vi "_io_write_with_OPC_synchro.vi"(4 "Send *ESR? at the end (T)":bool=TRUE, 5 "Attribute":T1={"Identifier"="", "Descriptive Name"="", "Data Type"=enum."Integer 32", "Command"="", "Access"=enum."Read/Write", "Range Table"="", "Read Callback"="", "Write Callback"="", "Supported Models"="", "Instrument Options"="", "Index"=0, "OPC Wait"=FALSE, "No Status Check"=FALSE, "Cache Only"=FALSE}, 7 "Timeout in (0 = OPC timeout)":i32, 8 "error in":errorcluster caption="error in (no error)", 10 "Write Command":string, 11 "VISA resource name":refnum<visa-resource-name>) -> (0 "error out":errorcluster, 2 "OPC Waited":bool, 3 "VISA resource name out":refnum<visa-resource-name>)   [LabVIEW 2020, in "Rohde&Schwarz RTx Oscilloscopes.lvlib" / "rsidr_core.lvlib"]
uses:
  rsidr_core.lvlib
  type_Attribute.ctl
  type_Attribute_Data_Type.ctl
  type_ReadWriteAccess.ctl
  whitespace.ctl
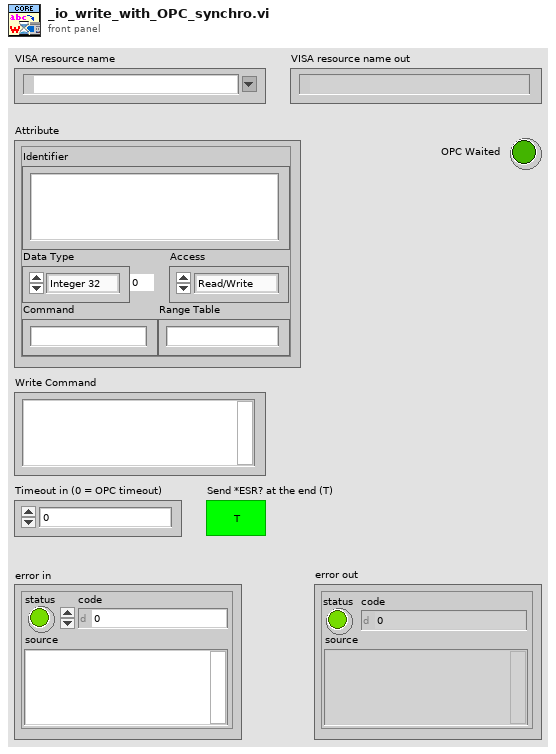
[diagram p1: front panel]
types:
  T1 = typedef "Rohde&Schwarz RTx Oscilloscopes.lvlib/rsidr_core.lvlib/type_Attribute.ctl" = cluster{"Identifier":string, "Descriptive Name":string, "Data Type":T2, "Command":string, "Access":T3, "Range Table":string, "Read Callback":string, "Write Callback":string, "Supported Models":string, "Instrument Options":string, "Index":i32, "OPC Wait":bool, "No Status Check":bool, "Cache Only":bool}
  T2 = typedef "Rohde&Schwarz RTx Oscilloscopes.lvlib/rsidr_core.lvlib/type_Attribute_Data_Type.ctl" = enum16{"Integer 32", "Double", "String", "Boolean", "None", "Integer 64", "RawString"}
  T3 = typedef "Rohde&Schwarz RTx Oscilloscopes.lvlib/rsidr_core.lvlib/type_ReadWriteAccess.ctl" = enum16{"Read Only", "Write Only", "Read/Write"}
  T4 = typedef "Rohde&Schwarz RTx Oscilloscopes.lvlib/rsidr_core.lvlib/type_Session_Data.ctl" = cluster{"IDN string":string, "Instrument FW":string, "Instr type":string, "Instr type for err. msg.":string, "Installed Options":string[], "Ignore Error Messages":string, "Logging params":variant, "OPC Timeout":i32, "VISA Timeout":i32, "STB Poll VISA Timeout":i32, "Additional Flags":i32, "Wait Before Read":i32, "Wait Before Write":i32, "Option String Flags":i32, "IO Segment Size":i64, "VISA Access Mode":T5, "Interface Type":T6, "OPC Wait Mode":T7, "Bin Float Number  Format":T8, "Bin Integer Number Format":T9, "Simulate":bool, "VXIcapable":bool, "Duplicate Session":bool, "Add LF to Write":bool, "Logging":bool, "Fast Sweep":bool, "Query Instrument Status":bool, "Check Range":bool, "Check Options":bool, "OPC-sync Attr Writes":bool, "OPC-sync Attr Queries":bool}
  T5 = typedef "Rohde&Schwarz RTx Oscilloscopes.lvlib/rsidr_core.lvlib/type_VisaAccessMode.ctl" = u16
  T6 = typedef "Rohde&Schwarz RTx Oscilloscopes.lvlib/rsidr_core.lvlib/type_InterfaceType.ctl" = enum16{"Unknown", "GPIB", "VXI", "GPIB_VXI", "ASRL", "PXI", "TCPIP", "USB", "SOCKET"}
  T7 = typedef "Rohde&Schwarz RTx Oscilloscopes.lvlib/rsidr_core.lvlib/type_OPC_Wait_Mode.ctl" = enum16{"STBpolling", "STBpollingSlow", "STBpollingSuperSlow", "ServiceRequest", "OPCquery"}
  T8 = typedef "Rohde&Schwarz RTx Oscilloscopes.lvlib/rsidr_core.lvlib/type_Binary_Float_Number_Format.ctl" = enum16{"Float_4_Bytes_Swapped", "Float_4_Bytes", "Double_8_Bytes_Swapped", "Double_8_Bytes"}
  T9 = typedef "Rohde&Schwarz RTx Oscilloscopes.lvlib/rsidr_core.lvlib/type_Binary_Integer_Number_Format.ctl" = enum16{"Int32_4_Bytes_Swapped", "Int32_4 Bytes", "Int16_2_Bytes_Swapped", "Int16_2_Bytes"}
  T10 = typedef "whitespace.ctl" = u16
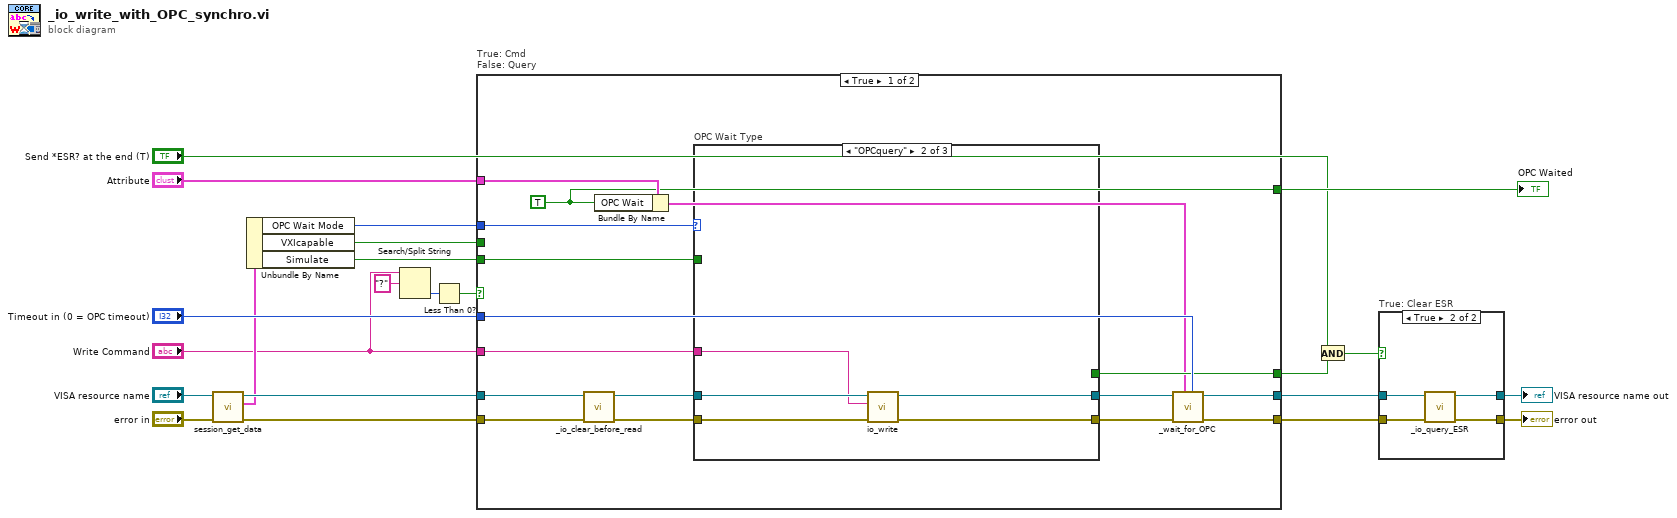
[diagram p0: block diagram]
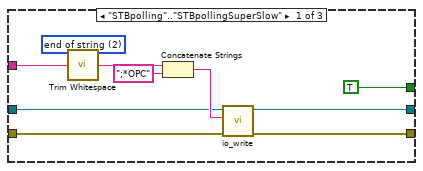
[diagram p2: hidden frame]
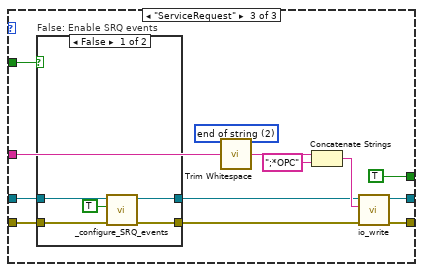
[diagram p3: hidden frame]
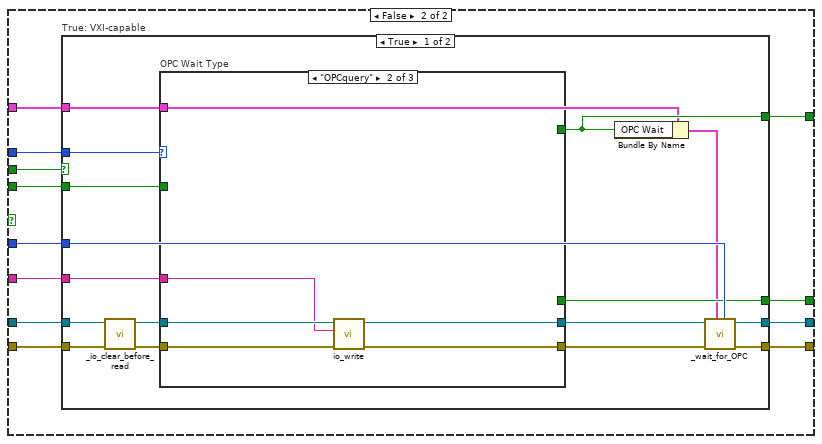
[diagram p5: hidden frame]
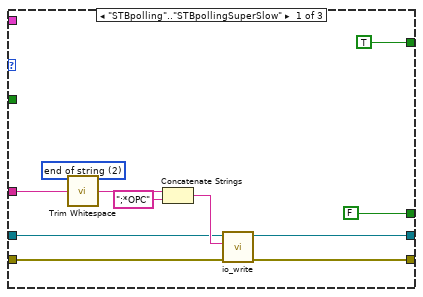
[diagram p6: hidden frame]
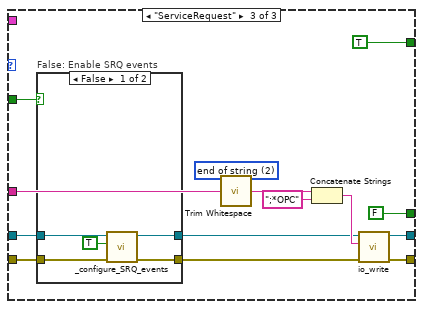
[diagram p7: hidden frame]
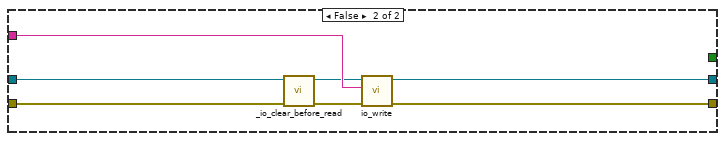
[diagram p9: hidden frame]
diagram:
  n1 = call "session_get_data.vi"("error in"="error in", "VISA resource name"="VISA resource name") -> ("error out"=w19:errorcluster, "Session User Data out"=w13:T4, "VISA resource name out"=w18:refnum<visa-resource-name>)  [unwired: 6 in, 1 out]
  n2 = Unbundle By Name(w13) -> ("OPC Wait Mode"=w10:T7, "VXIcapable"=w11:bool, "Simulate"=w9:bool)
  n3 = Search/Split String(string="Write Command", search string/char (-)="?") -> (offset of match=w6:i32)  [unwired: 1 in, 2 out]
  n4 = Less Than 0?(x=w6) -> (x < 0?=w4:bool)
  n5 = case "True: Cmd\nFalse: Query" shown="True" w4 {
    tunnel: "Timeout in (0 = OPC timeout)" -> [w38 w85]
    tunnel: w19 -> [w37 w84]
    tunnel: w18 -> [w36 w83]
    tunnel: [w35 w82] -> w2
    tunnel: [w30 w77] -> w17
    tunnel: [w29 w76] -> w16
    tunnel: "Attribute" -> [w34 w81]
    tunnel: w11 -> [_ w75]
    tunnel: w10 -> [w33 w80]
    tunnel: w9 -> [w32 w79]
    tunnel: [w23 w74] -> w8
    tunnel: "Write Command" -> [w31 w78]
    frame True {
      w23 = TRUE ("Flag: OPC Wait")
      n6 = call "_io_clear_before_read.vi"("error in"=w37, "VISA resource name"=w36) -> ("error out"=w28:errorcluster, "VISA resource name out"=w27:refnum<visa-resource-name>)  [unwired: 8 in]
      n7 = Bundle By Name(cluster=w34, "OPC Wait"=w23) -> (w24:T1)
      n8 = case "OPC Wait Type" shown="\"OPCquery\"" w33 {
        tunnel: w28 -> [w42 w53 w61]
        tunnel: w27 -> [w43 w52 w60]
        tunnel: w31 -> [w45 w51 w58]
        tunnel: [w41 w50 w56] -> w26
        tunnel: [w40 w49 w55] -> w25
        tunnel: w32 -> [_ _ w62]
        tunnel: [TRUE _ TRUE] -> w35
        frame "STBpolling".."STBpollingSuperSlow" {
          w46 = T10 2 items=["both", "start of string", "end of string"] ("location (both)")
          n9 = call "Trim Whitespace.vi"("string"=w45, "location (both)"=w46) -> ("trimmed string"=w44:string)
          n10 = Concatenate Strings(w44, ";*OPC" ("string")) -> (w48:string)
          n11 = call "io_write.vi"("error in"=w42, "write buffer"=w48, "VISA resource name"=w43) -> ("error out"=w41:errorcluster, "VISA resource name out"=w40:refnum<visa-resource-name>)  [unwired: 7 in]
        }
        frame "OPCquery" {
          (unwired) TRUE
          n12 = call "io_write.vi"("error in"=w53, "write buffer"=w51, "VISA resource name"=w52) -> ("error out"=w50:errorcluster, "VISA resource name out"=w49:refnum<visa-resource-name>)  [unwired: 7 in]
        }
        frame "ServiceRequest" {
          w59 = T10 2 items=["both", "start of string", "end of string"] ("location (both)")
          n13 = case "False: Enable SRQ events" shown="False" w62 {
            tunnel: w61 -> [w71 w73]
            tunnel: w60 -> [w70 w72]
            tunnel: [w69 w73] -> w64
            tunnel: [w68 w72] -> w63
            frame False {
              n14 = call "_configure_SRQ_events.vi"("error in"=w71, "Enable"=TRUE, "VISA resource name"=w70) -> ("error out"=w69:errorcluster, "VISA resource name out"=w68:refnum<visa-resource-name>)  [unwired: 7 in]
            }
            frame True {
            }
          }
          n15 = call "Trim Whitespace.vi"("string"=w58, "location (both)"=w59) -> ("trimmed string"=w57:string)
          n16 = Concatenate Strings(w57, ";*OPC" ("string")) -> (w66:string)
          n17 = call "io_write.vi"("error in"=w64, "write buffer"=w66, "VISA resource name"=w63) -> ("error out"=w56:errorcluster, "VISA resource name out"=w55:refnum<visa-resource-name>)  [unwired: 7 in]
        }
      }
      n18 = call "_wait_for_OPC.vi"("Timeout in (0 = OPC timeout)"=w38, "Attribute"=w24, "error in"=w26, "VISA resource name"=w25) -> ("error out"=w30:errorcluster, "VISA resource name out"=w29:refnum<visa-resource-name>)  [unwired: 6 in]
    }
    frame False {
      n19 = case "True: VXI-capable" shown="True" w75 {
        tunnel: w85 -> [w101 _]
        tunnel: w84 -> [w100 w145]
        tunnel: w83 -> [w99 w144]
        tunnel: [w98 _] -> w82
        tunnel: w81 -> [w87 _]
        tunnel: w80 -> [w97 _]
        tunnel: w79 -> [w96 _]
        tunnel: w78 -> [w95 w143]
        tunnel: [w94 w139] -> w77
        tunnel: [w93 w140] -> w76
        tunnel: [w88 _] -> w74
        frame True {
          n20 = call "_io_clear_before_read.vi"("error in"=w100, "VISA resource name"=w99) -> ("error out"=w92:errorcluster, "VISA resource name out"=w91:refnum<visa-resource-name>)  [unwired: 8 in]
          n21 = case "OPC Wait Type" shown="\"OPCquery\"" w97 {
            tunnel: w92 -> [w106 w117 w126]
            tunnel: w91 -> [w107 w116 w125]
            tunnel: w95 -> [w109 w115 w123]
            tunnel: [w105 w114 w121] -> w90
            tunnel: [w104 w113 w120] -> w89
            tunnel: w96 -> [_ _ w127]
            tunnel: [FALSE _ FALSE] -> w98
            tunnel: w87 -> [_ _ _]
            tunnel: [TRUE ("Flag: OPC Wait") _ TRUE ("Flag: OPC Wait")] -> w88
            frame "STBpolling".."STBpollingSuperSlow" {
              w110 = T10 2 items=["both", "start of string", "end of string"] ("location (both)")
              n22 = call "Trim Whitespace.vi"("string"=w109, "location (both)"=w110) -> ("trimmed string"=w108:string)
              n23 = Concatenate Strings(w108, ";*OPC" ("string")) -> (w112:string)
              n24 = call "io_write.vi"("error in"=w106, "write buffer"=w112, "VISA resource name"=w107) -> ("error out"=w105:errorcluster, "VISA resource name out"=w104:refnum<visa-resource-name>)  [unwired: 7 in]
            }
            frame "OPCquery" {
              (unwired) TRUE
              n25 = call "io_write.vi"("error in"=w117, "write buffer"=w115, "VISA resource name"=w116) -> ("error out"=w114:errorcluster, "VISA resource name out"=w113:refnum<visa-resource-name>)  [unwired: 7 in]
            }
            frame "ServiceRequest" {
              w124 = T10 2 items=["both", "start of string", "end of string"] ("location (both)")
              n26 = case "False: Enable SRQ events" shown="False" w127 {
                tunnel: w126 -> [w136 w138]
                tunnel: w125 -> [w135 w137]
                tunnel: [w134 w138] -> w129
                tunnel: [w133 w137] -> w128
                frame False {
                  n27 = call "_configure_SRQ_events.vi"("error in"=w136, "Enable"=TRUE, "VISA resource name"=w135) -> ("error out"=w134:errorcluster, "VISA resource name out"=w133:refnum<visa-resource-name>)  [unwired: 7 in]
                }
                frame True {
                }
              }
              n28 = call "Trim Whitespace.vi"("string"=w123, "location (both)"=w124) -> ("trimmed string"=w122:string)
              n29 = Concatenate Strings(w122, ";*OPC" ("string")) -> (w131:string)
              n30 = call "io_write.vi"("error in"=w129, "write buffer"=w131, "VISA resource name"=w128) -> ("error out"=w121:errorcluster, "VISA resource name out"=w120:refnum<visa-resource-name>)  [unwired: 7 in]
            }
          }
          n31 = Bundle By Name(cluster=w87, "OPC Wait"=w88) -> (w86:T1)
          n32 = call "_wait_for_OPC.vi"("Timeout in (0 = OPC timeout)"=w101, "Attribute"=w86, "error in"=w90, "VISA resource name"=w89) -> ("error out"=w94:errorcluster, "VISA resource name out"=w93:refnum<visa-resource-name>)  [unwired: 6 in]
        }
        frame False {
          n33 = call "_io_clear_before_read.vi"("error in"=w145, "VISA resource name"=w144) -> ("error out"=w142:errorcluster, "VISA resource name out"=w141:refnum<visa-resource-name>)  [unwired: 8 in]
          n34 = call "io_write.vi"("error in"=w142, "write buffer"=w143, "VISA resource name"=w141) -> ("error out"=w139:errorcluster, "VISA resource name out"=w140:refnum<visa-resource-name>)  [unwired: 7 in]
        }
      }
    }
  }
  "OPC Waited" <- w8
  n35 = And(x="Send *ESR? at the end (T)", y=w2) -> (x .and. y?=w1:bool)
  n36 = case "True: Clear ESR" shown="True" w1 {
    tunnel: w17 -> [w147 w151]
    tunnel: w16 -> [w146 w150]
    tunnel: [w147 w149] -> w15
    tunnel: [w146 w148] -> w14
    frame False {
    }
    frame True {
      n37 = call "_io_query_ESR.vi"("error in"=w151, "VISA resource name"=w150) -> ("error out"=w149:errorcluster, "VISA resource name out"=w148:refnum<visa-resource-name>)  [unwired: 7 in, 1 out]
    }
  }
  "VISA resource name out" <- w14
  "error out" <- w15
